vi "Test_WriteValue_TransportClosed_WriteError.vi"(8 "error in (no error)":errorcluster, 11 "TestCase in":refnum<class "TestEventTransport.lvclass">) -> (0 "error out":errorcluster, 3 "TestCase out":refnum<class "TestEventTransport.lvclass">)   [LabVIEW 2017, in "TestEventTransport.lvclass"]
uses:
  TestEventTransport.lvclass
  Source/Concrete/EventTransport/EventTransport.lvclass/EventTransport.ctl
  Source/Concrete/EventTransport/EventTransport.lvclass
  C:/Git/composed-transport/Source/ITransport/ITransport.lvclass
  Source/ITransport/ITransport.lvclass
panel:
  out "Return Error":errorcluster
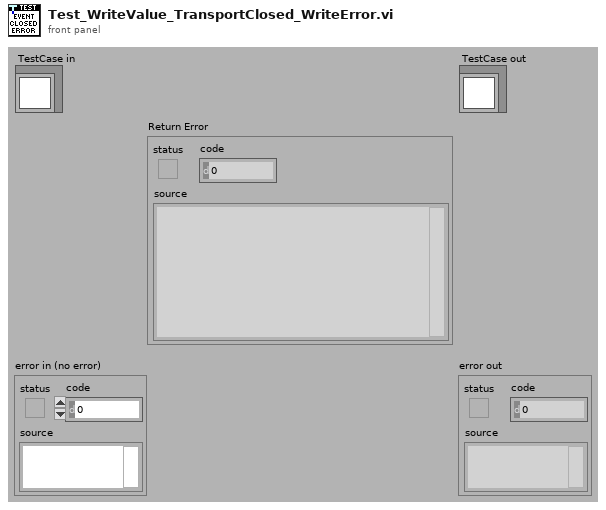
[diagram p1: front panel]
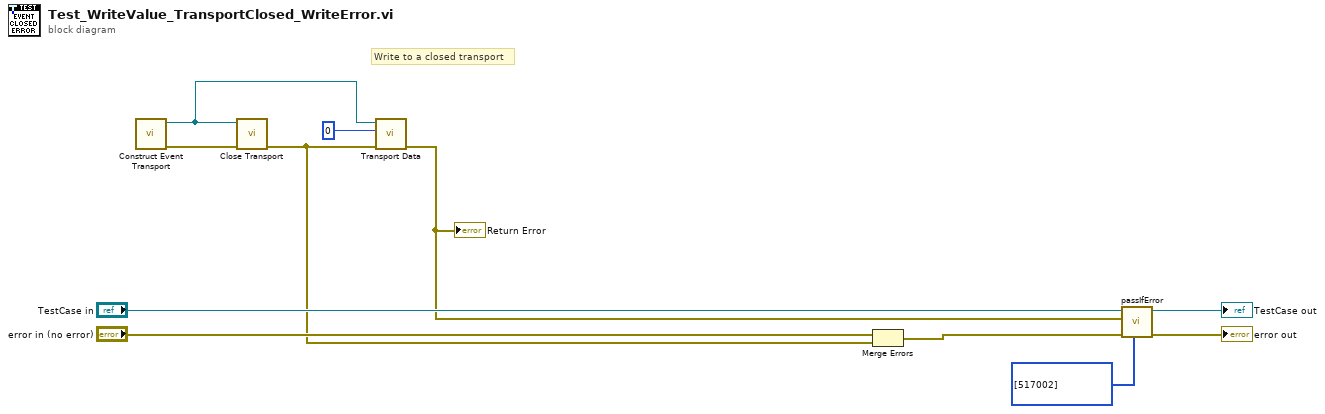
[diagram p0: block diagram]
diagram:
  # "Write to a closed transport"
  n1 = call "Construct Event Transport.vi"() -> ("error out"=w3:errorcluster, "EventTransport"=w1:refnum<class "EventTransport.lvclass">)  [unwired: 9 in, 1 out]
  n2 = call-dynamic "Close Transport.vi"("error in (no error)"=w3, "EventTransport"=w1) -> ("error out"=w2:errorcluster)  [unwired: 9 in]
  n3 = call "Transport Data.vi"("error in (no error)"=w2, "Value"=0, "ITransport in"=w1) -> ("error out"=w5:errorcluster)  [unwired: 7 in, 1 out]
  "Return Error" <- w5
  n4 = Merge Errors("error in (no error)", w2) -> (w7:errorcluster)
  n5 = call-dynamic "passIfError.vi"("passing error codes (default = any error code)"=i32[] [517002], "error in (no error)"=w7, "error"=w5, "TestCase in"="TestCase in") -> ("error out"=→"error out":errorcluster, "TestCase out"=→"TestCase out":refnum<class "TestEventTransport.lvclass">)  [unwired: 6 in]
